vi "area_fit_old.vi"(10 "Parameters Fit":T1, 11 "FWHM":dbl=4.0 format="%#_13g") -> (2 "Err. Area":dbl, 3 "Area":dbl)   [LabVIEW 2020]
uses:
  <vilib>/gmath/statdist.llb/Normal CDF.vi
  <vilib>/gmath/NI_Gmath.lvlib
panel:
  out "x-y":dbl
  out "Area Brutale":dbl
  out "Area Totale":dbl
  out "x-fwhm":dbl
  out "x+fwhm":dbl
  out "percentuale":dbl
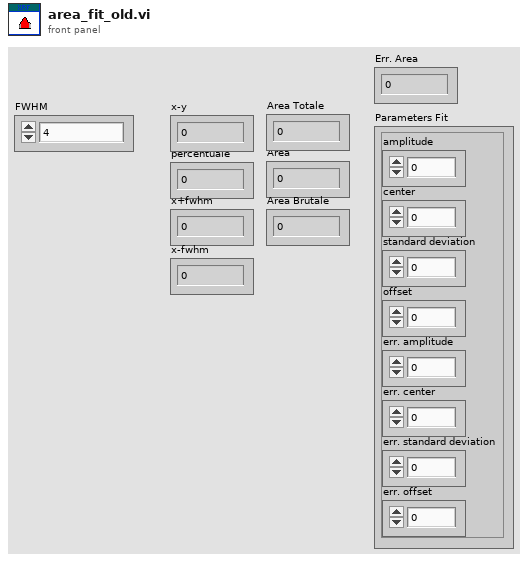
[diagram p1: front panel]
types:
  T1 = cluster{"amplitude":dbl, "center":dbl, "standard deviation":dbl, "offset":dbl, "err. amplitude":dbl, "err. center":dbl, "err. standard deviation":dbl, "err. offset":dbl}
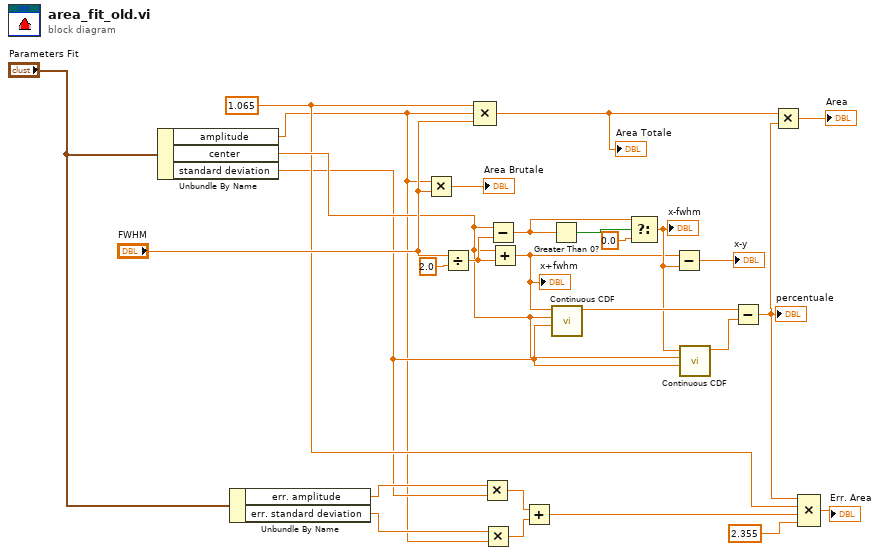
[diagram p0: block diagram]
diagram:
  w11 = 1.065 ("value")
  n1 = Unbundle By Name("Parameters Fit") -> ("amplitude"=w2:dbl, "center"=w15:dbl, "standard deviation"=w3:dbl)
  n2 = Unbundle By Name("Parameters Fit") -> ("err. amplitude"=w5:dbl, "err. standard deviation"=w4:dbl)
  n3 = Multiply(x=w2, y="FWHM") -> (x*y=→"Area Brutale":dbl)
  n4 = Divide(x="FWHM", y=2.0 ("x")) -> (x/y=w20:dbl)
  n5 = Compound Arithmetic op=MULTIPLY(w11, w2, "FWHM") -> (w13:dbl)
  "Area Totale" <- w13
  n6 = Multiply(x=w5, y=w3) -> (x*y=w8:dbl)
  n7 = Multiply(x=w4, y=w2) -> (x*y=w9:dbl)
  n8 = Subtract(x=w15, y=w20) -> (x-y=w24:dbl)
  n9 = Add(x=w15, y=w20) -> (x+y=w17:dbl)
  "x+fwhm" <- w17
  n10 = Add(x=w8, y=w9) -> (x+y=w7:dbl)
  n11 = Greater Than 0?(x=w24) -> (x > 0?=w25:bool)
  n12 = call-poly <vilib>:"Continuous CDF.vi"("std"=w3, "mean"=w15, "x"=w17) -> ("cdf(x)"=w27:dbl)  [unwired: 7 in, 1 out]
  n13 = Select(t=w24, s=w25, f=0.0) -> (s? t:f=w18:dbl)
  "x-fwhm" <- w18
  n14 = Subtract(x=w17, y=w18) -> (x-y=→"x-y":dbl)
  n15 = call-poly <vilib>:"Continuous CDF.vi"("std"=w3, "mean"=w15, "x"=w18) -> ("cdf(x)"=w26:dbl)  [unwired: 7 in, 1 out]
  n16 = Subtract(x=w27, y=w26) -> (x-y=w12:dbl)
  "percentuale" <- w12
  n17 = Multiply(x=w13, y=w12) -> (x*y=→"Area":dbl)
  n18 = Compound Arithmetic op=MULTIPLY(w12, w11, w7, 2.355 ("y")) -> (→"Err. Area":dbl)
